vi "BRig_dataMTrig_SolenoidCal_I_R.vi"() -> (2 "output_SolenoidCal_I_R":i32)   [LabVIEW 2014]
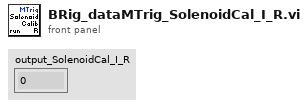
[diagram p1: front panel]
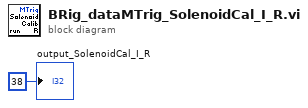
[diagram p0: block diagram]
diagram:
  "output_SolenoidCal_I_R" <- 38 ("output_iBlock")
